vi "STOP.vi"(11 "Pump_1AI_1DO_2DI in":refnum<class "NeedleValve.lvclass">) -> (3 "Pump_1AI_1DO_2DI out":refnum<class "NeedleValve.lvclass">)   [LabVIEW 2019, in "NeedleValve.lvclass"]
uses:
  NeedleValve.lvclass
  NeedleValve.lvclass/NeedleValve.ctl
  TypeDef/Needle Valve State.ctl
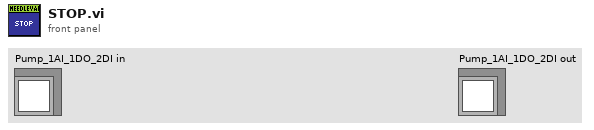
[diagram p1: front panel]
types:
  T1 = typedef "Needle Valve State.ctl" = enum16{"IDLE", "OPENING", "CLOSING", "STOP"}
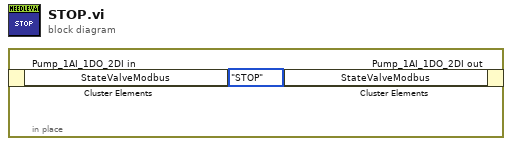
[diagram p0: block diagram]
diagram:
  n1 = in-place {
    n2 = in-place-cluster #1("Pump_1AI_1DO_2DI in") -> ()  [unwired: 1 out]
    n3 = in-place-cluster #1("StateValveModbus"=Needle_Valve_State."STOP") -> (→"Pump_1AI_1DO_2DI out":refnum<class "NeedleValve.lvclass">)
  }
